vi "Runtime Config.vi"(10 "Configuration 2":T1={"Primary Filter"="<NO FILTER>", "Secondary Filter"="<NO FILTER>", "Slit Mask"="<NO MASK>", "Grating"="<NO GRATING>", "CS Target"=0.0, "GS Target"=0.0, "Coll Focus"=1000, "Camera Focus"=0, "Name"="", "User"="", "Date"="", "Comment"="", "use Flexure Comp?"=TRUE, "Select Mode:"=0} {"Select Mode:" items=["Custom", "Imaging", "300 All", "600 UV", "600 Blue", "600 Mid", "600 Red", "1200 m0", "1200 m1", "1200 m2", "1200 m3", "1200 m4", "1200 m5", "1200 m6", "1200 m7", "1200 RESOLVE", "400 m1", "400 m2", "930 m1", "930 m2", "930 m3", "930 m4", "930 m5", "930 m6", "400WD", "930TP", "400Fermi", "400Padgett", "400Lewis", "400Crotts", "600BLee", "600RLee", "400WW", "ZZ Ceti Red", "ZZ Ceti Blue"]}, 11 "Configuration":T1={"Primary Filter"="<NO FILTER>", "Secondary Filter"="<NO FILTER>", "Slit Mask"="<NO MASK>", "Grating"="<NO GRATING>", "CS Target"=0.0, "GS Target"=0.0, "Coll Focus"=1000, "Camera Focus"=0, "Name"="", "User"="", "Date"="", "Comment"="", "use Flexure Comp?"=TRUE, "Select Mode:"=0} {"Select Mode:" items=["Custom", "Imaging", "300 All", "600 UV", "600 Blue", "600 Mid", "600 Red", "1200 m0", "1200 m1", "1200 m2", "1200 m3", "1200 m4", "1200 m5", "1200 m6", "1200 m7", "1200 RESOLVE", "400 m1", "400 m2", "930 m1", "930 m2", "930 m3", "930 m4", "930 m5", "930 m6", "400WD", "930TP", "400Fermi", "400Padgett", "400Lewis", "400Crotts", "600BLee", "600RLee", "400WW", "ZZ Ceti Red", "ZZ Ceti Blue"]}) -> (3 "time":dbl)   [LabVIEW 2015]
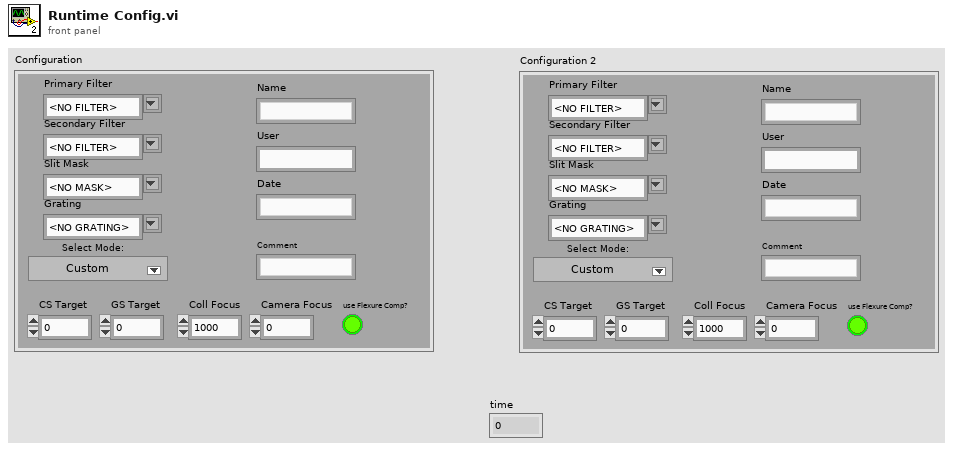
[diagram p1: front panel]
types:
  T1 = cluster{"Primary Filter":string, "Secondary Filter":string, "Slit Mask":string, "Grating":string, "CS Target":dbl, "GS Target":dbl, "Coll Focus":i32, "Camera Focus":i32, "Name":string, "User":string, "Date":string, "Comment":string, "use Flexure Comp?":bool, "Select Mode:":u16}
  T2 = cluster{"Primary Filter":bool, "Secondary Filter":bool, "Slit Mask":bool, "Grating":bool, "CS Target":bool, "GS Target":bool, "Coll Focus":bool, "Camera Focus":bool, "Name":bool, "User":bool, "Date":bool, "Comment":bool, "use Flexure Comp?":bool, "Select Mode:":bool}
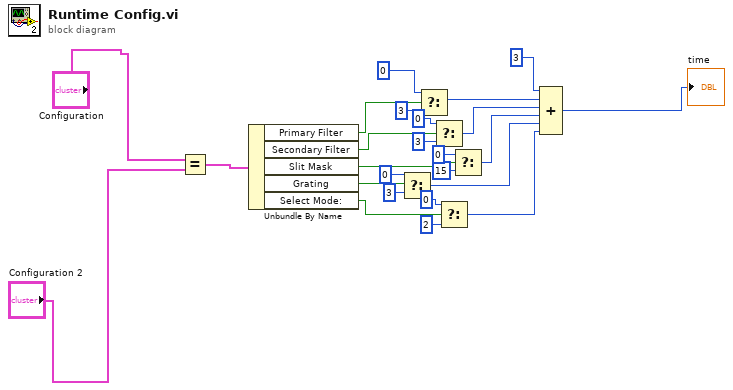
[diagram p0: block diagram]
diagram:
  n1 = Equal?(x="Configuration", y="Configuration 2") -> (x = y?=w23:T2)
  n2 = Unbundle By Name(w23) -> ("Primary Filter"=w22:bool, "Secondary Filter"=w21:bool, "Slit Mask"=w20:bool, "Grating"=w19:bool, "Select Mode:"=w18:bool)
  n3 = Select(t=0, s=w19, f=3) -> (s? t:f=w13:i32)
  n4 = Select(t=0, s=w22, f=3) -> (s? t:f=w16:i32)
  n5 = Select(t=0, s=w21, f=3) -> (s? t:f=w15:i32)
  n6 = Select(t=0, s=w18, f=2) -> (s? t:f=w12:i32)
  n7 = Select(t=0, s=w20, f=15) -> (s? t:f=w14:i32)
  n8 = Compound Arithmetic op=ADD(3, w16, w15, w14, w13, w12) -> (→"time":i32)
